vi "ManipEnd.vi"() -> (0 "Error Out":errorcluster, 1 "Advance Trigger":bool)   [LabVIEW 2020]
doc: "Stops the subsystem sequencer.\n\nParameters: None"
uses:
  autonomousinfo.vi
  drivercommands.vi
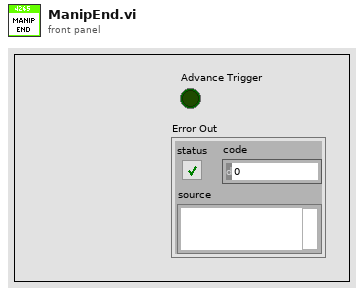
[diagram p1: front panel]
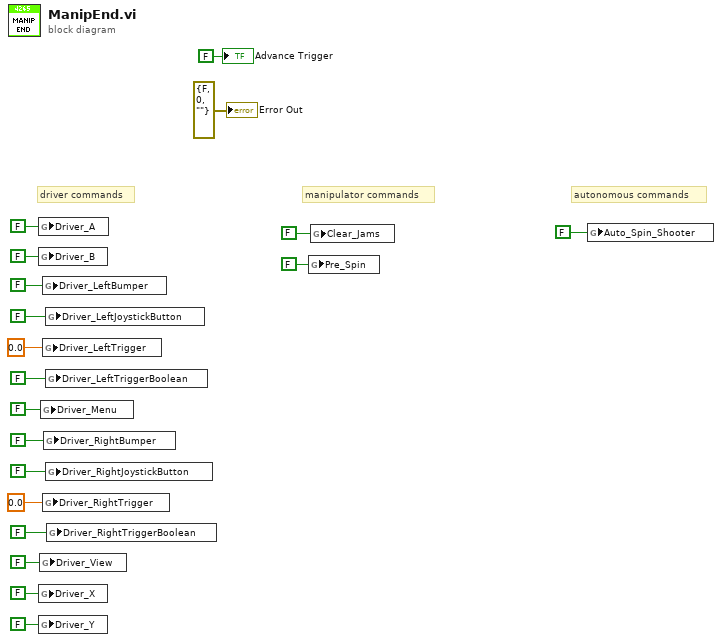
[diagram p0: block diagram]
diagram:
  # "manipulator commands"
  # "driver commands"
  # "autonomous commands"
  n1 = global write "drivercommands.vi" "Driver_A"(FALSE ("Driver_A")) -> ()
  n2 = global write "drivercommands.vi" "Driver_B"(FALSE ("Driver_B")) -> ()
  n3 = global write "drivercommands.vi" "Driver_X"(FALSE ("Driver_X")) -> ()
  n4 = global write "drivercommands.vi" "Driver_Y"(FALSE ("Driver_Y")) -> ()
  n5 = global write "drivercommands.vi" "Driver_View"(FALSE ("Driver_View")) -> ()
  n6 = global write "drivercommands.vi" "Driver_Menu"(FALSE ("Driver_Menu")) -> ()
  n7 = global write "drivercommands.vi" "Driver_LeftBumper"(FALSE ("Driver_LeftBumper")) -> ()
  n8 = global write "drivercommands.vi" "Driver_LeftTrigger"(0.0 ("Driver_LeftTrigger")) -> ()
  n9 = global write "drivercommands.vi" "Driver_RightTrigger"(0.0 ("Driver_RightTrigger")) -> ()
  n10 = global write "drivercommands.vi" "Driver_RightBumper"(FALSE ("Driver_RightBumper")) -> ()
  n11 = global write "drivercommands.vi" "Driver_LeftJoystickButton"(FALSE ("Driver_LeftJoystickButton")) -> ()
  n12 = global write "drivercommands.vi" "Driver_LeftTriggerBoolean"(FALSE ("Driver_LeftTriggerBoolean")) -> ()
  n13 = global write "drivercommands.vi" "Driver_RightJoystickButton"(FALSE ("Driver_RightJoystickButton")) -> ()
  n14 = global write "drivercommands.vi" "Driver_RightTriggerBoolean"(FALSE ("Driver_RightTriggerBoolean")) -> ()
  n15 = global write "drivercommands.vi" "Pre_Spin"(FALSE ("Clear_Jams")) -> ()
  n16 = global write "drivercommands.vi" "Clear_Jams"(FALSE ("Clear_Jams")) -> ()
  n17 = global write "autonomousinfo.vi" "Auto_Spin_Shooter"(FALSE ("Auto_Spin_Shooter")) -> ()
  "Advance Trigger" <- FALSE ("Advance Trigger")
  "Error Out" <- errorcluster {"status"=FALSE, "code"=0, "source"=""} ("error constant")
